vi "BASE.Device.Disconnect.vi"(8 "error in (no error)":errorcluster, 10 "Timeout (5000 ms)":i32, 11 "Device.Simulation in":refnum<class "Device.Simulation.lvclass">) -> (0 "error out":errorcluster, 3 "Device.Simulation out":refnum<class "Device.Simulation.lvclass">)   [LabVIEW 2019, in "Device.Simulation.lvlib" / "Device.Simulation.lvclass"]
uses:
  Device.Simulation.lvclass
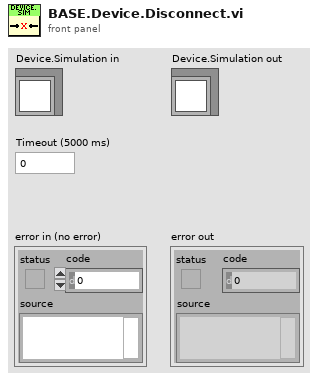
[diagram p1: front panel]
types:
  T1 = typedef "Device.Simulation.lvlib/Device.Simulation.lvclass/config--cluster.ctl" = cluster{"Name":string, "Time to Connect (ms)":u32, "Time to Check Connection (ms)":u32, "Time to Disconnect (ms)":u32, "Time to Read State (ms)":u32}
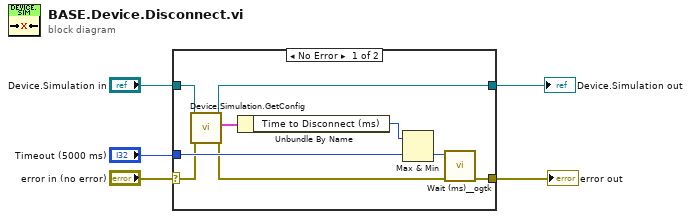
[diagram p0: block diagram]
diagram:
  n1 = case shown="No Error" "error in (no error)" {
    selector: "error in (no error)" -> [w8 w16]
    tunnel: [w14 w16] -> w4
    tunnel: "Device.Simulation in" -> [w10 w15]
    tunnel: [w9 w15] -> w3
    tunnel: "Timeout (5000 ms)" -> [w11 _]
    frame No Error {
      n2 = call "Device.Simulation.GetConfig.vi"("error in (no error)"=w8, "Device.Simulation in"=w10) -> ("error out"=w7:errorcluster, "config"=w6:T1, "Device.Simulation out"=w9:refnum<class "Device.Simulation.lvclass">)  [unwired: 7 in]
      n3 = Unbundle By Name(w6) -> ("Time to Disconnect (ms)"=w12:u32)
      n4 = Max & Min(x=w12, y=w11) -> (min(x,y)=w13:u32)  [unwired: 1 out]
      n5 = call <userlib>:"Wait (ms)__ogtk.vi"("error in (no error)"=w7, "milliseconds to wait"=w13) -> ("error out"=w14:errorcluster)  [unwired: 8 in, 1 out]
    }
    frame Error {
    }
  }
  "error out" <- w4
  "Device.Simulation out" <- w3
